vi "Screenshot Flash.vi"(8 "Error In":errorcluster, 11 "Image Data":T1) -> (0 "Error Out":errorcluster, 3 "new picture":picture)   [LabVIEW 2020]
uses:
  <vilib>/picture/picture.llb/imagedata.ctl
  c082308f-ba6d-4afb-af71-4bd932213d53.vi
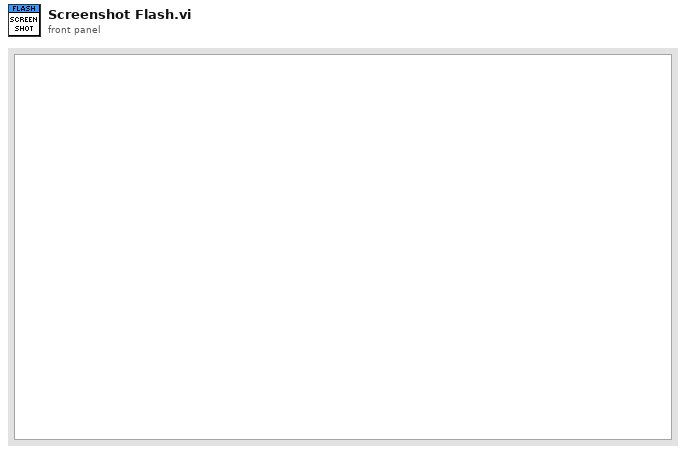
[diagram p1: front panel]
types:
  T1 = typedef "imagedata.ctl" = cluster{"image type":i32, "image depth":i32, "image":u8[], "mask":u8[], "colors":u32[], "Rectangle":cluster{"left":i16, "top":i16, "right":i16, "bottom":i16}}
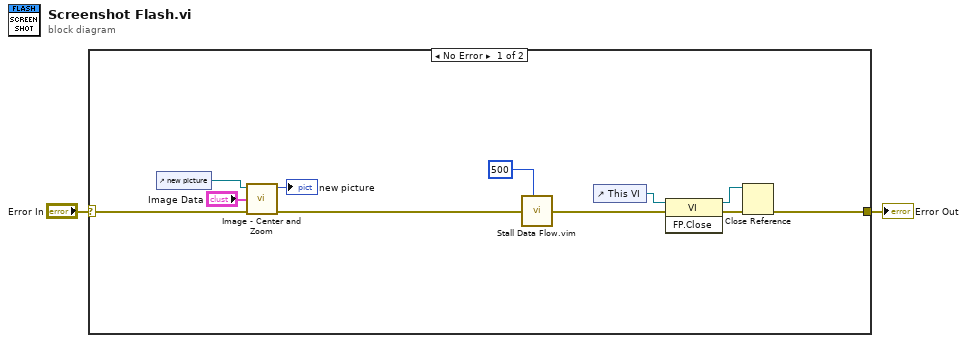
[diagram p0: block diagram]
diagram:
  n1 = case shown="No Error" "Error In" {
    selector: "Error In" -> [w11 w14]
    tunnel: [w12 w14] -> w2
    frame No Error {
      n2 = control-ref of="new picture"() -> (w7:refnum<vi>)
      n3 = call "Image - Center and Zoom.vi"("Error In"=w11, "Image Data"="Image Data", "Pict Refnum"=w7) -> ("Error Out"=w5:errorcluster, "new picture"=→"new picture":picture)  [unwired: 6 in, 1 out]
      n4 = call "Stall Data Flow.vim"("value in"=w5, "milliseconds to wait"=u32 500) -> ("value out"=w4:errorcluster)  [unwired: 1 out]
      n5 = control-ref of="This VI"() -> (w9:refnum<vi>)
      n6 = invoke class="VI" method="FP.Close"(reference=w9, error in=w4) -> (reference out=w10:refnum<vi>, error out=w13:errorcluster)  [unwired: 1 in, 1 out]
      n7 = Close Reference(reference=w10, error in (no error)=w13) -> (error out=w12:errorcluster)
    }
    frame Error {
    }
  }
  "Error Out" <- w2
